vi "InitCSMs.vi"(8 "error in":errorcluster, 11 "testcase-CSMResponse.lvclass in":refnum<class "testcase-CSMResponse.lvclass">) -> (0 "error out":errorcluster, 3 "testcase-CSMResponse.lvclass out":refnum<class "testcase-CSMResponse.lvclass">)   [LabVIEW 2017, in "testcase-CSMResponse.lvclass"]
uses:
  testcase-CSMResponse.lvclass
  testcase-CSMResponse.lvclass/testcase-CSMResponse.ctl
  CSM/Chain1.vi
  CSM/Chain2.vi
  CSM/Chain3.vi
  <vilib>/AppBuilder/AB_API_Simple/Build (path).vi
  CSM/CSM-Testcase.lvlib
  src/user.lib/_NEVSTOP/Communicable State Machine(CSM)/Communicable State Machine.lvlib
  <vilib>/AppBuilder/AB_API_Simple/NI_App_Builder_API.lvlib
panel:
  out "Waited (ms)":u32
  out "CSMs Left":string[](array[string])
  out "CSMs":string[](array[string])
  out "Generated files":path[](array[path])
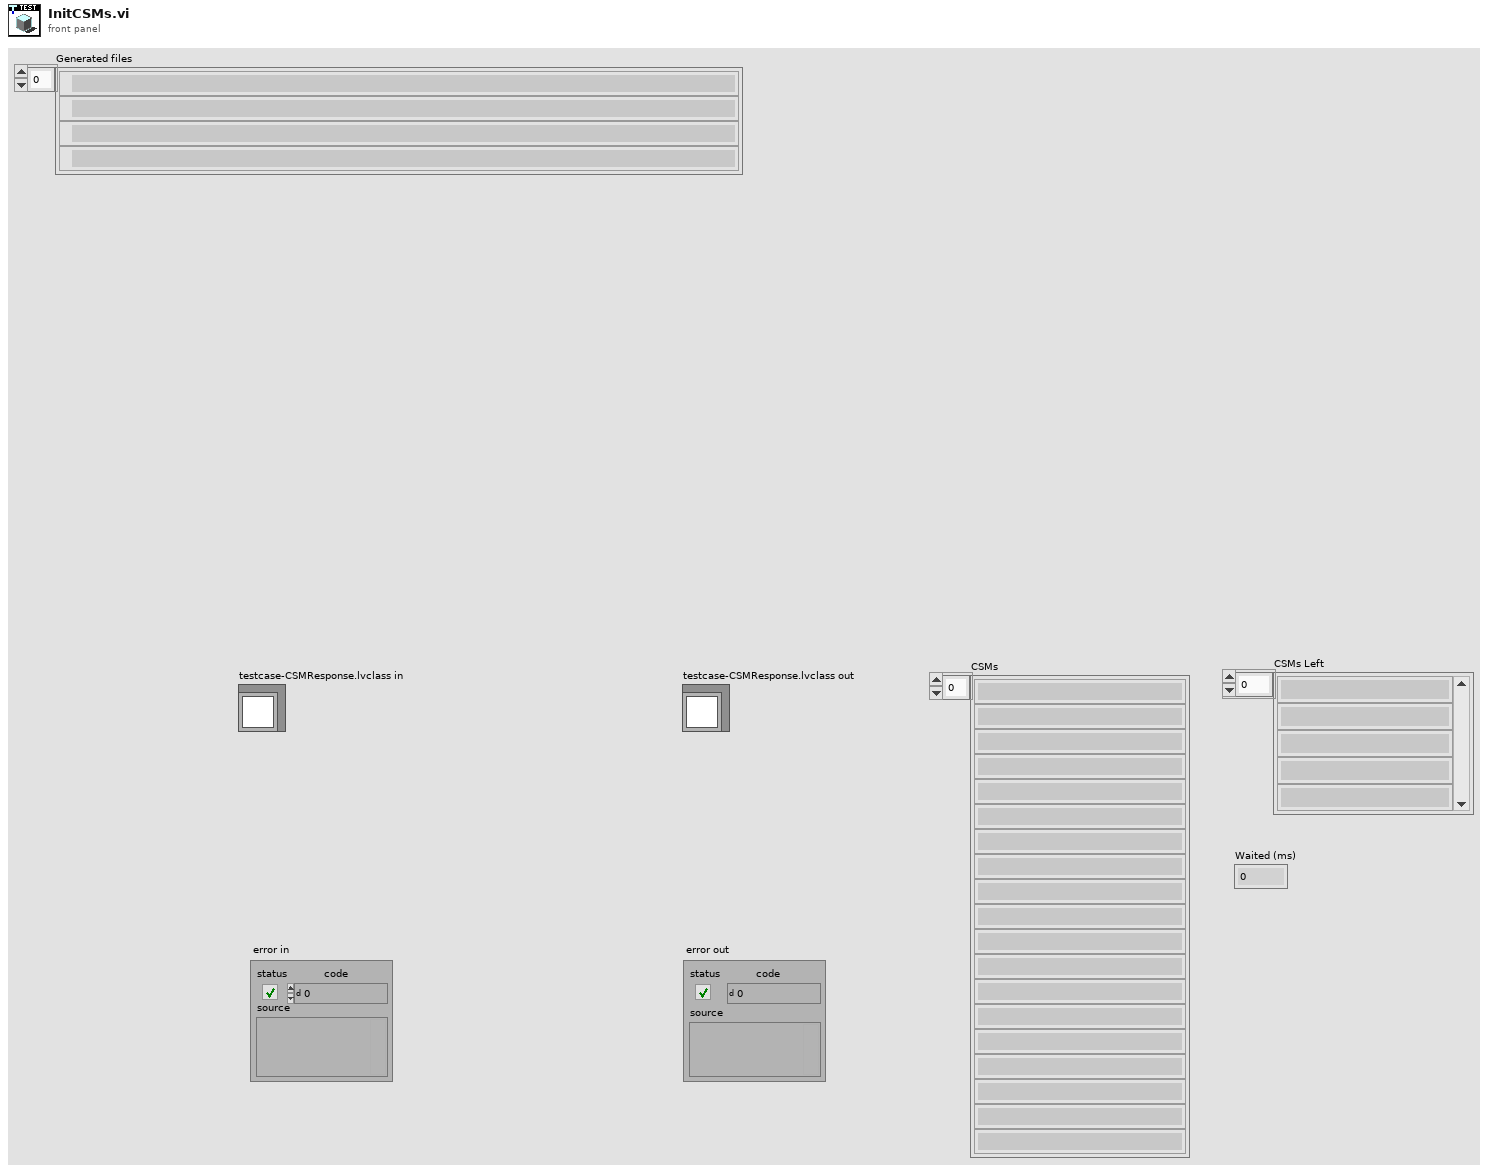
[diagram p1: front panel]
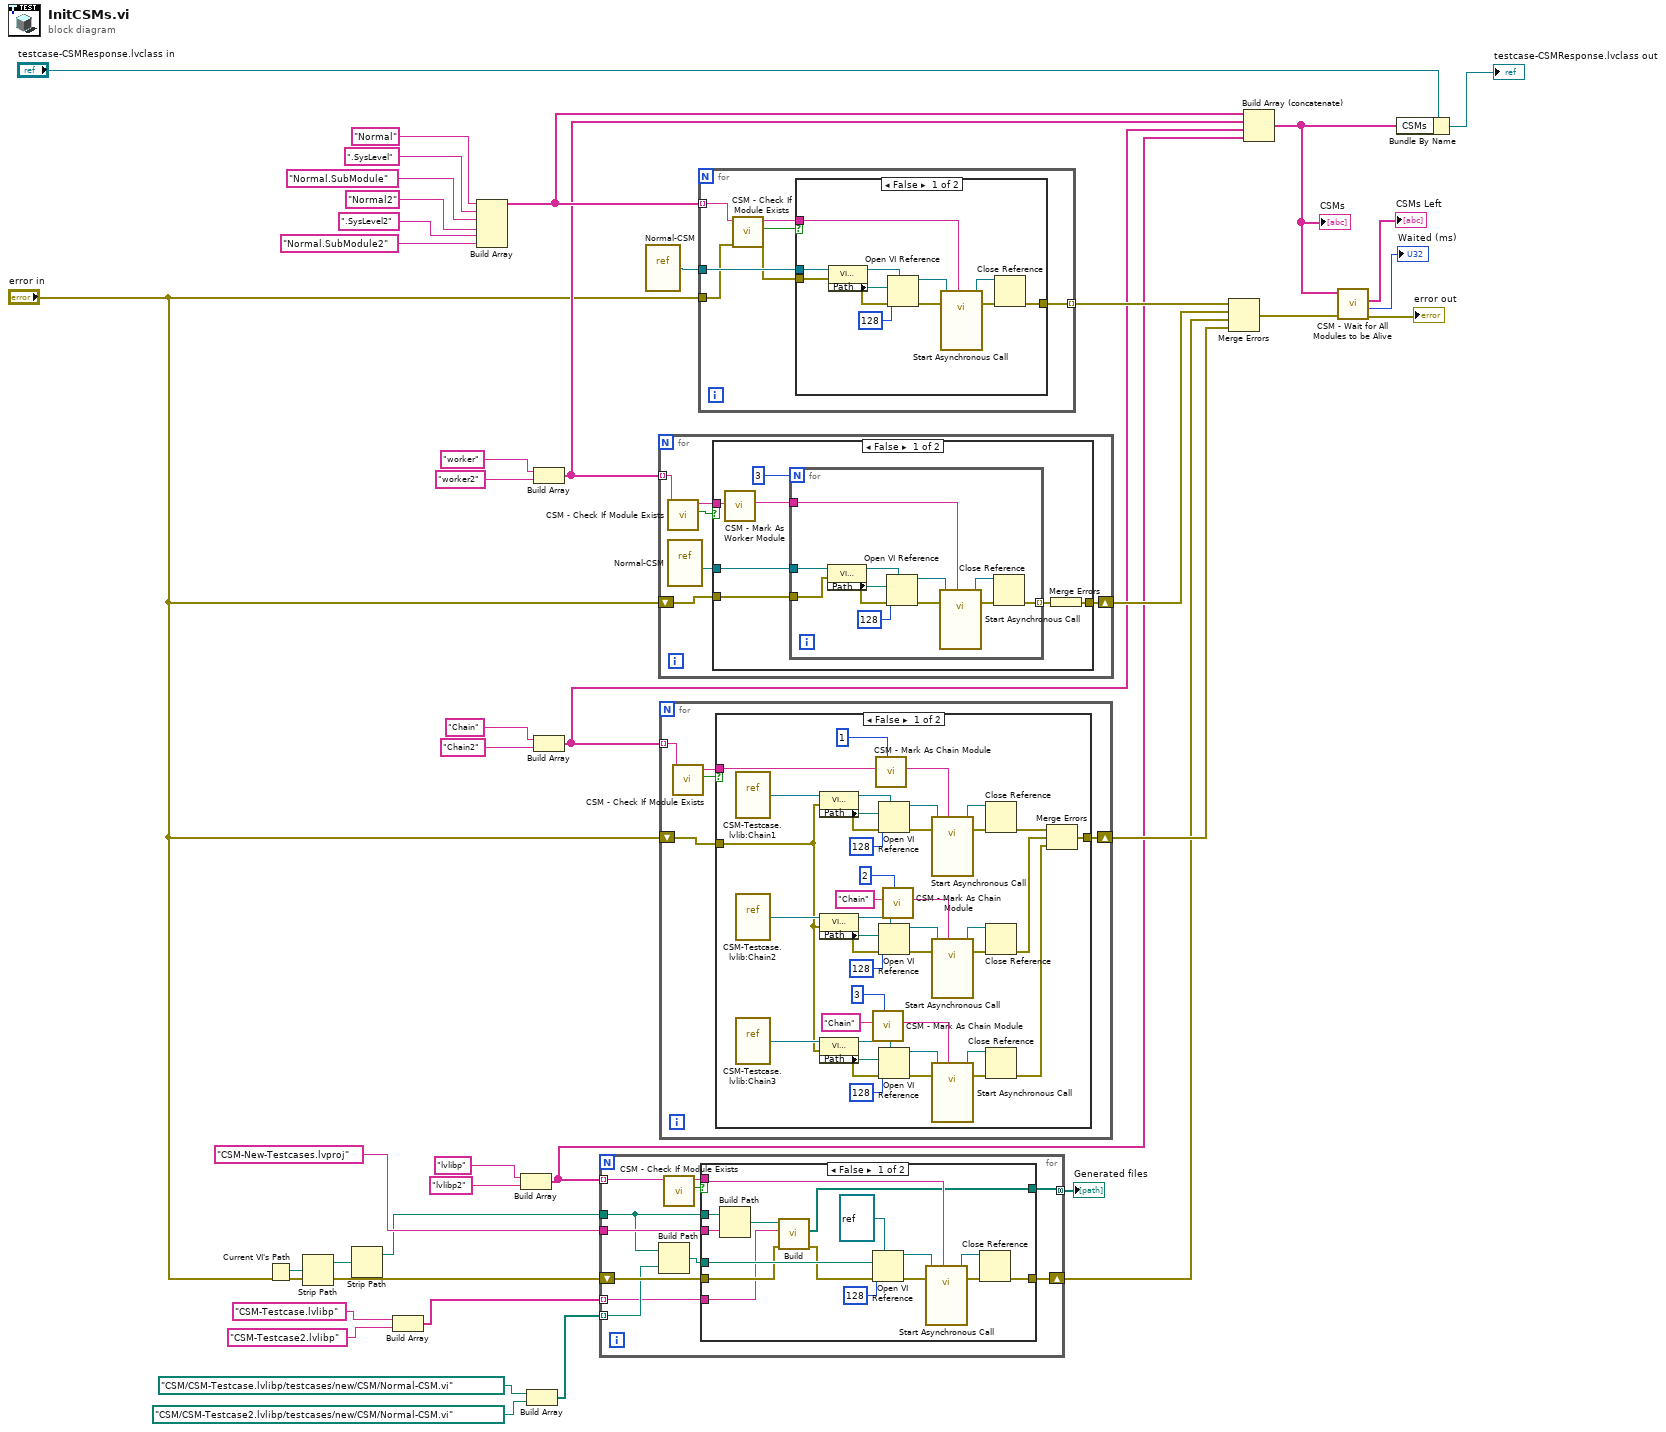
[diagram p0: block diagram]
diagram:
  n1 = Current VI's Path() -> (path=w36:path)
  n2 = Strip Path(path=w36) -> (stripped path=w37:path)  [unwired: 1 out]
  n3 = Strip Path(path=w37) -> (stripped path=w38:path)  [unwired: 1 out]
  n4 = Build Array("CSM-Testcase.lvlibp" ("Name of build specification (if empty: build all)"), "CSM-Testcase2.lvlibp" ("Name of build specification (if empty: build all)")) -> (w10:string[])
  n5 = Build Array("Normal" ("Name (\"\" to Use UUID)"), ".SysLevel" ("Name (\"\" to Use UUID)"), "Normal.SubModule" ("Name (\"\" to Use UUID)"), "Normal2" ("Name (\"\" to Use UUID)"), ".SysLevel2" ("Name (\"\" to Use UUID)"), "Normal.SubModule2" ("Name (\"\" to Use UUID)")) -> (w32:string[])
  n6 = Build Array("lvlibp" ("Name (\"\" to Use UUID)"), "lvlibp2" ("Name (\"\" to Use UUID)")) -> (w16:string[])
  n7 = Build Array(path "CSM/CSM-Testcase.lvlibp/testcases/new/CSM/Normal-CSM.vi" ("vi path"), path "CSM/CSM-Testcase2.lvlibp/testcases/new/CSM/Normal-CSM.vi" ("vi path")) -> (w13:path[])
  n8 = Build Array("worker" ("Name (\"\" to Use UUID)"), "worker2" ("Name (\"\" to Use UUID)")) -> (w22:string[])
  n9 = Build Array("Chain" ("Name (\"\" to Use UUID)"), "Chain2" ("Name (\"\" to Use UUID)")) -> (w19:string[])
  n10 = for {
    tunnel: "CSM-New-Testcases.lvproj" ("name or relative path") -> [w49]
    tunnel: w38 -> [w44]
    shift-right: [w48] -> w35
    shift-left: "error in" -> [w50]
    tunnel: w16 -> [w46] mode=indexing
    tunnel: w13 -> [w45] mode=indexing
    tunnel: w10 -> [w42] mode=indexing
    tunnel: [w41] -> w9 mode=concatenating
    n11 = Build Path(base path=w44, name or relative path=w45) -> (appended path=w43:path)
    n12 = call "CSM - Check If Module Exists.vi"("CSM Name"=w46) -> ("Exist?"=w51:bool, "CSM Name (Dup)"=w47:string)  [unwired: 8 in, 1 out]
    n13 = case shown="False" w51 {
      tunnel: [w67 w68] -> w48
      tunnel: w43 -> [w60 _]
      tunnel: w44 -> [w59 _]
      tunnel: w49 -> [w57 _]
      tunnel: w47 -> [w56 _]
      tunnel: w50 -> [w55 w68]
      tunnel: w42 -> [w53 _]
      tunnel: [w52 _] -> w41
      frame False {
        n14 = Build Path(base path=w59, name or relative path=w57) -> (appended path=w58:path)
        n15 = call-poly <vilib>:"Build.vi"("error in (no error)"=w55, "Name of build specification (if empty: build all)"=w53, "Path to project"=w58) -> ("error out"=w54:errorcluster, "Generated files"=w52:path[])  [unwired: 7 in]
        n16 = Open VI Reference(type specifier VI Refnum (for type only)=refnum<vi> refnum ("reference out"), vi path=w60, options=128, error in (no error)=w54) -> (vi reference=w63:refnum<vi>, error out=w65:errorcluster)  [unwired: 2 in]
        n17 = call-by-ref "Start Asynchronous Call"(reference=w63, error in=w65, "Name (\"\" to Use UUID)"=w56) -> (reference out=w62:refnum<vi>, error out=w64:errorcluster)  [unwired: 11 in]
        n18 = Close Reference(reference=w62, error in (no error)=w64) -> (error out=w67:errorcluster)
      }
      frame True {
      }
    }
  }
  "Generated files" <- w9
  n19 = vi-ref "Normal-CSM.vi"() -> (w28:refnum<vi>)
  n20 = for {
    shift-right: [w71] -> w34
    shift-left: "error in" -> [w74]
    tunnel: w22 -> [w69] mode=indexing
    n21 = call "CSM - Check If Module Exists.vi"("CSM Name"=w69) -> ("Exist?"=w73:bool, "CSM Name (Dup)"=w72:string)  [unwired: 8 in, 1 out]
    n22 = vi-ref "Normal-CSM.vi"() -> (w70:refnum<vi>)
    n23 = case shown="False" w73 {
      tunnel: w70 -> [w81 _]
      tunnel: [w75 w94] -> w71
      tunnel: w74 -> [w77 w94]
      tunnel: w72 -> [w76 _]
      frame False {
        n24 = call "CSM - Mark As Worker Module.vi"("CSM Name"=w76) -> ("CSM Name (Marked As Worker)"=w78:string)  [unwired: 9 in]
        n25 = for {
          N: 3 -> [_]
          tunnel: w81 -> [w85]
          tunnel: w78 -> [w84]
          tunnel: [w83] -> w79 mode=indexing
          tunnel: w77 -> [w82]
          n26 = property class="VI (strict)"(reference=w85, error in=w82) -> (reference out=w91:refnum<vi>, error out=w89:errorcluster, "Path"=w88:path)
          n27 = Open VI Reference(type specifier VI Refnum (for type only)=w91, vi path=w88, options=128, error in (no error)=w89) -> (vi reference=w87:refnum<vi>, error out=w92:errorcluster)  [unwired: 2 in]
          n28 = call-by-ref "Start Asynchronous Call"(reference=w87, error in=w92, "Name (\"\" to Use UUID)"=w84) -> (reference out=w86:refnum<vi>, error out=w90:errorcluster)  [unwired: 11 in]
          n29 = Close Reference(reference=w86, error in (no error)=w90) -> (error out=w83:errorcluster)
        }
        n30 = Merge Errors(w79) -> (w75:errorcluster)
      }
      frame True {
      }
    }
  }
  n31 = for {
    shift-right: [w97] -> w40
    shift-left: "error in" -> [w99]
    tunnel: w19 -> [w95] mode=indexing
    n32 = call "CSM - Check If Module Exists.vi"("CSM Name"=w95) -> ("Exist?"=w98:bool, "CSM Name (Dup)"=w96:string)  [unwired: 8 in, 1 out]
    n33 = case shown="False" w98 {
      tunnel: [w102 w141] -> w97
      tunnel: w99 -> [w101 w141]
      tunnel: w96 -> [w100 _]
      frame False {
        n34 = vi-ref "CSM-Testcase.lvlib:Chain1.vi"() -> (w140:refnum<vi>)
        n35 = vi-ref "CSM-Testcase.lvlib:Chain2.vi"() -> (w123:refnum<vi>)
        n36 = vi-ref "CSM-Testcase.lvlib:Chain3.vi"() -> (w120:refnum<vi>)
        n37 = property class="VI (strict)"(reference=w140, error in=w101) -> (reference out=w137:refnum<vi>, error out=w135:errorcluster, "Path"=w134:path)
        n38 = property class="VI (strict)"(reference=w123, error in=w101) -> (reference out=w126:refnum<vi>, error out=w128:errorcluster, "Path"=w129:path)
        n39 = property class="VI (strict)"(reference=w120, error in=w101) -> (reference out=w117:refnum<vi>, error out=w115:errorcluster, "Path"=w114:path)
        n40 = call "CSM - Mark As Chain Module.vi"("Order"=3, "CSM Name"="Chain" ("Name (\"\" to Use UUID)")) -> ("CSM Name (Marked As Chain)"=w108:string)  [unwired: 8 in]
        n41 = call "CSM - Mark As Chain Module.vi"("Order"=1, "CSM Name"=w100) -> ("CSM Name (Marked As Chain)"=w106:string)  [unwired: 8 in]
        n42 = Open VI Reference(type specifier VI Refnum (for type only)=w137, vi path=w134, options=128, error in (no error)=w135) -> (vi reference=w133:refnum<vi>, error out=w138:errorcluster)  [unwired: 2 in]
        n43 = Open VI Reference(type specifier VI Refnum (for type only)=w126, vi path=w129, options=128, error in (no error)=w128) -> (vi reference=w130:refnum<vi>, error out=w125:errorcluster)  [unwired: 2 in]
        n44 = Open VI Reference(type specifier VI Refnum (for type only)=w117, vi path=w114, options=128, error in (no error)=w115) -> (vi reference=w113:refnum<vi>, error out=w118:errorcluster)  [unwired: 2 in]
        n45 = call "CSM - Mark As Chain Module.vi"("Order"=2, "CSM Name"="Chain" ("Name (\"\" to Use UUID)")) -> ("CSM Name (Marked As Chain)"=w107:string)  [unwired: 8 in]
        n46 = call-by-ref "Start Asynchronous Call"(reference=w133, error in=w138, "Name (\"\" to Use UUID)"=w106) -> (reference out=w132:refnum<vi>, error out=w136:errorcluster)  [unwired: 11 in]
        n47 = call-by-ref "Start Asynchronous Call"(reference=w130, error in=w125, "Name (\"\" to Use UUID)"=w107) -> (reference out=w131:refnum<vi>, error out=w127:errorcluster)  [unwired: 11 in]
        n48 = call-by-ref "Start Asynchronous Call"(reference=w113, error in=w118, "Name (\"\" to Use UUID)"=w108) -> (reference out=w112:refnum<vi>, error out=w116:errorcluster)  [unwired: 11 in]
        n49 = Close Reference(reference=w132, error in (no error)=w136) -> (error out=w111:errorcluster)
        n50 = Close Reference(reference=w131, error in (no error)=w127) -> (error out=w110:errorcluster)
        n51 = Close Reference(reference=w112, error in (no error)=w116) -> (error out=w109:errorcluster)
        n52 = Merge Errors(w111, w110, w109) -> (w102:errorcluster)
      }
      frame True {
      }
    }
  }
  n53 = for {
    tunnel: w28 -> [w148]
    tunnel: w32 -> [w144] mode=indexing
    tunnel: [w147] -> w33 mode=indexing
    tunnel: "error in" -> [w146]
    n54 = call "CSM - Check If Module Exists.vi"("Error In"=w146, "CSM Name"=w144) -> ("error out"=w145:errorcluster, "Exist?"=w142:bool, "CSM Name (Dup)"=w143:string)  [unwired: 7 in]
    n55 = case shown="False" w142 {
      tunnel: w148 -> [w152 _]
      tunnel: [w151 w161] -> w147
      tunnel: w145 -> [w150 w161]
      tunnel: w143 -> [w149 _]
      frame False {
        n56 = property class="VI (strict)"(reference=w152, error in=w150) -> (reference out=w158:refnum<vi>, error out=w156:errorcluster, "Path"=w155:path)
        n57 = Open VI Reference(type specifier VI Refnum (for type only)=w158, vi path=w155, options=128, error in (no error)=w156) -> (vi reference=w154:refnum<vi>, error out=w159:errorcluster)  [unwired: 2 in]
        n58 = call-by-ref "Start Asynchronous Call"(reference=w154, error in=w159, "Name (\"\" to Use UUID)"=w149) -> (reference out=w153:refnum<vi>, error out=w157:errorcluster)  [unwired: 11 in]
        n59 = Close Reference(reference=w153, error in (no error)=w157) -> (error out=w151:errorcluster)
      }
      frame True {
      }
    }
  }
  n60 = Merge Errors(w33, w34, w35, w40) -> (w5:errorcluster)
  n61 = Build Array (concatenate)(w32, w22, w19, w16) -> (w3:string[])
  "CSMs" <- w3
  n62 = call "CSM - Wait for All Modules to be Alive.vi"("Error In"=w5, "CSM Names"=w3) -> ("error out"=→"error out":errorcluster, "Waited (ms)"=→"Waited (ms)":u32, "CSMs Left"=→"CSMs Left":string[])  [unwired: 7 in]
  n63 = Bundle By Name(cluster="testcase-CSMResponse.lvclass in", "CSMs"=w3) -> (→"testcase-CSMResponse.lvclass out":refnum<class "testcase-CSMResponse.lvclass">)
